vi "ReadIonWeightImg.vi"() -> (3 "ion weight":dbl[][](array[numeric]))   [LabVIEW 2019]
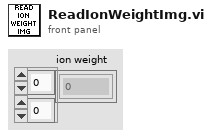
[diagram p1: front panel]
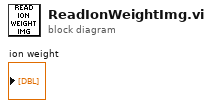
[diagram p0: block diagram]
diagram:
